vi "Get All Channel Names from List.vi"(8 "error in (no error)":errorcluster, 11 "Pairing Tab Refs":T1) -> (0 "error out":errorcluster, 2 "Channel Names":string[](array[string]))   [LabVIEW 2015, in "E2E Tag Exchange editor node.lvclass"]
uses:
  E2E Tag Exchange editor node.lvclass
  Tag Exchange Tab References.ctl
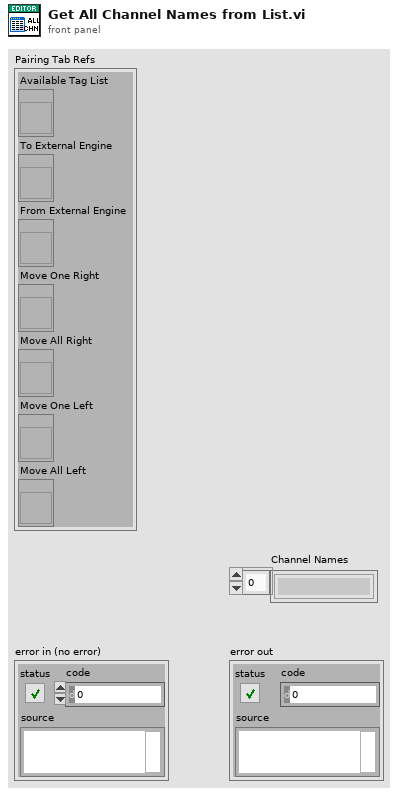
[diagram p1: front panel]
types:
  T1 = typedef "E2E Tag Exchange editor node.lvclass/Tag Exchange Tab References.ctl" = cluster{"Available Tag List":refnum<vi>, "To External Engine":refnum<vi>, "From External Engine":refnum<vi>, "Move One Right":refnum<vi>, "Move All Right":refnum<vi>, "Move One Left":refnum<vi>, "Move All Left":refnum<vi>}
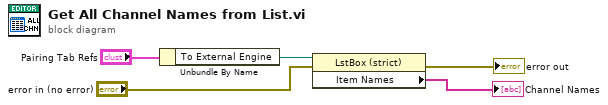
[diagram p0: block diagram]
diagram:
  n1 = Unbundle By Name("Pairing Tab Refs") -> ("To External Engine"=w4:refnum<vi>)
  n2 = property class="LstBox (strict)"(reference=w4, error in="error in (no error)") -> (error out=→"error out":errorcluster, "Item Names"=→"Channel Names":string[])  [unwired: 1 out]
